vi "ALTS-2015 LV2GBL Robot FIFO Queue.vi"(7 "Enum":enum16{"Init", "Enqueue", "Dequeue", "Destroy"}(ring), 8 "error in (no error)":errorcluster, 11 "Serial Details In":T1 {"Height" format="%.2g"}) -> (0 "error out":errorcluster, 2 "timed out?":bool, 3 "Serial Details Out":T1 {"Height" format="%.2g"})   [LabVIEW 2013]
uses:
  Controls/ALTS-2015 Serial Details.ctl
  Controls/ALTS-2015 Station Cluster.ctl
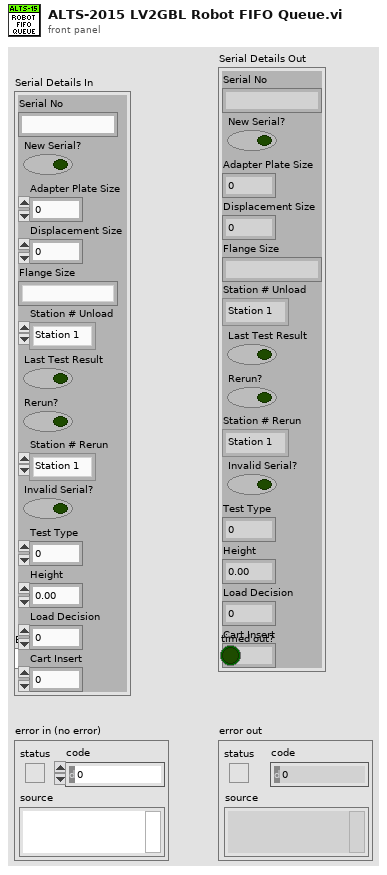
[diagram p1: front panel]
types:
  T1 = typedef "ALTS-2015 Serial Details.ctl" = cluster{"Serial No":string, "New Serial?":bool, "Adapter Plate Size":i32, "Displacement Size":i32, "Flange Size":string, "Station # Unload":T2, "Last Test Result":bool, "Rerun?":bool, "Station # Rerun":T2, "Invalid Serial?":bool, "Test Type":i32, "Height":dbl, "Load Decision":i32, "Cart Insert":i32}
  T2 = typedef "ALTS-2015 Station Cluster.ctl" = enum16{"Station 1", "Station 2", "Station 3", "Station 4"}
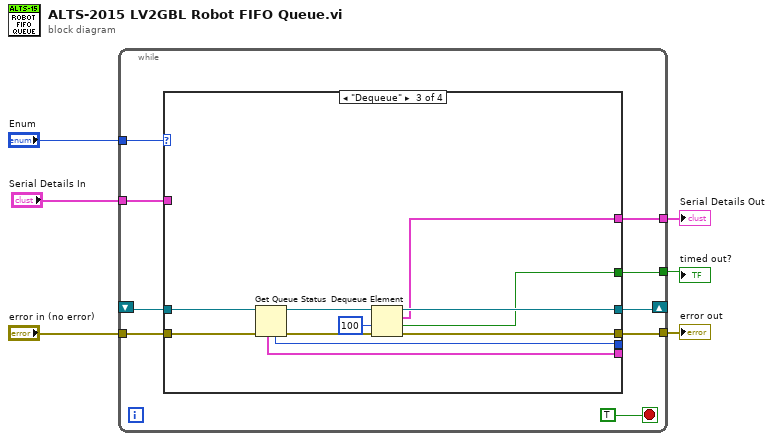
[diagram p0: block diagram]
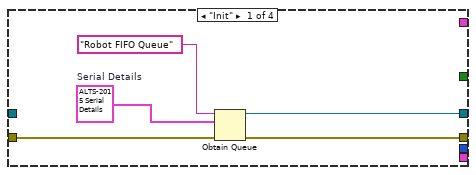
[diagram p2: hidden frame]
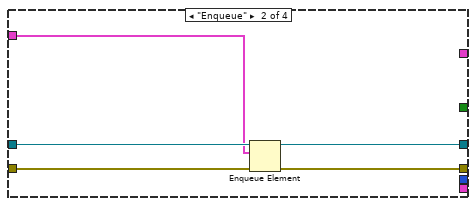
[diagram p3: hidden frame]
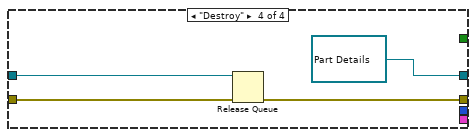
[diagram p4: hidden frame]
diagram:
  n1 = while {
    tunnel: "Enum" -> [w15]
    tunnel: "error in (no error)" -> [w13]
    tunnel: [w12] -> w4
    shift-right: [w11] -> _
    shift-left: _ -> [w9]
    tunnel: "Serial Details In" -> [w10]
    tunnel: [w8] -> w2
    tunnel: [w7] -> w1
    stop <- TRUE stop-if-true
    n2 = case shown="\"Dequeue\"" w15 {
      tunnel: w13 -> [w20 w25 w36 w40]
      tunnel: [w19 w22 w34 w38] -> w12
      tunnel: [w18 w23 w33 refnum<queue> refnum ("queue out")] -> w11
      tunnel: w10 -> [_ w21 _ _]
      tunnel: w9 -> [_ w24 w29 w39]
      tunnel: [_ _ w32 _] -> w8
      tunnel: [_ _ w31 _] -> w7
      tunnel: [_ _ w27 _] -> _
      tunnel: [_ _ w26 _] -> _
      frame "Init" {
        w17 = T1 {"Serial No"="", "New Serial?"=FALSE, "Adapter Plate Size"=0, "Displacement Size"=0, "Flange Size"="", "Station # Unload"=enum."Station 1", "Last Test Result"=FALSE, "Rerun?"=FALSE, "Station # Rerun"=enum."Station 1", "Invalid Serial?"=FALSE, "Test Type"=0, "Height"=0.0, "Load Decision"=0, "Cart Insert"=0}  # Serial Details
        n3 = Obtain Queue(name (unnamed)="Robot FIFO Queue", element data type=w17, error in (no error)=w20) -> (queue out=w18:refnum<queue>, error out=w19:errorcluster)  [unwired: 2 in, 1 out]
      }
      frame "Enqueue" {
        n4 = Enqueue Element(queue=w24, element=w21, error in (no error)=w25) -> (queue out=w23:refnum<queue>, error out=w22:errorcluster)  [unwired: 1 in, 1 out]
      }
      frame "Dequeue" {
        n5 = Get Queue Status(queue=w29, error in (no error)=w36) -> (queue out=w28:refnum<queue>, error out=w30:errorcluster, # elements in queue=w27:i32, elements=w26:T1[])  [unwired: 1 in, 4 out]
        n6 = Dequeue Element(queue=w28, timeout in ms (-1)=100, error in (no error)=w30) -> (queue out=w33:refnum<queue>, element=w32:T1, timed out?=w31:bool, error out=w34:errorcluster)
      }
      frame "Destroy" {
        n7 = Release Queue(queue=w39, error in (no error)=w40) -> (error out=w38:errorcluster)  [unwired: 1 in, 2 out]
      }
    }
  }
  "error out" <- w4
  "Serial Details Out" <- w2
  "timed out?" <- w1
